vi "6.vi"() -> ()   [LabVIEW 2017]
panel:
  out "字符串":string
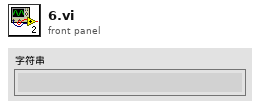
[diagram p1: front panel]
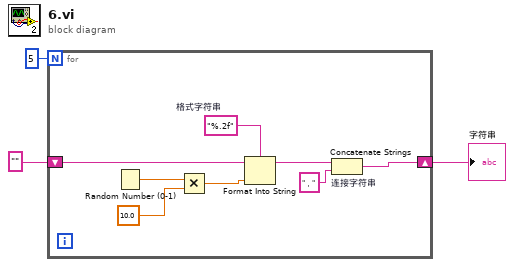
[diagram p0: block diagram]
diagram:
  n1 = for {
    N: 5 -> [_]
    shift-right: [w4] -> w1
    shift-left: "" -> [w7]
    w8 = "%.2f"  # 格式字符串
    n2 = Random Number (0-1)() -> (number: 0 to 1=w11:dbl)
    n3 = Multiply(x=w11, y=10.0) -> (x*y=w9:dbl)
    n4 = Format Into String(format string=w8, initial string=w7, w9) -> (resulting string=w6:string)  [unwired: 1 in, 1 out]
    n5 = Concatenate Strings "连接字符串"(w6, "，" ("字符串")) -> (w4:string)
  }
  "字符串" <- w1
